vi "Startup.vi"(6 "LabVIEW Web Service":refnum<class "Web Service.lvclass">) -> ()   [LabVIEW 2017]
uses:
  <vilib>/wsapi/Web Service.lvclass
  <vilib>/NI_Real-Time Target Support.lvlib
panel:
  # "Use the web service input terminal to call the VIs on the Service subpalette of the Web Services palette. Do not remove it from the connector pane unless you don't need access to the palette."
  # "Any additional terminals added to the connector pane of a startup VI will be ignored."
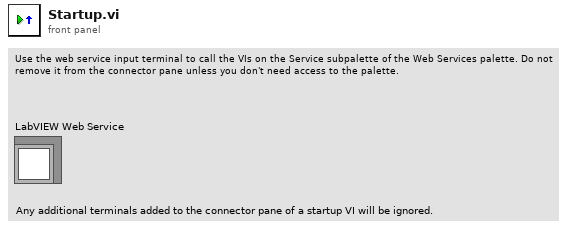
[diagram p1: front panel]
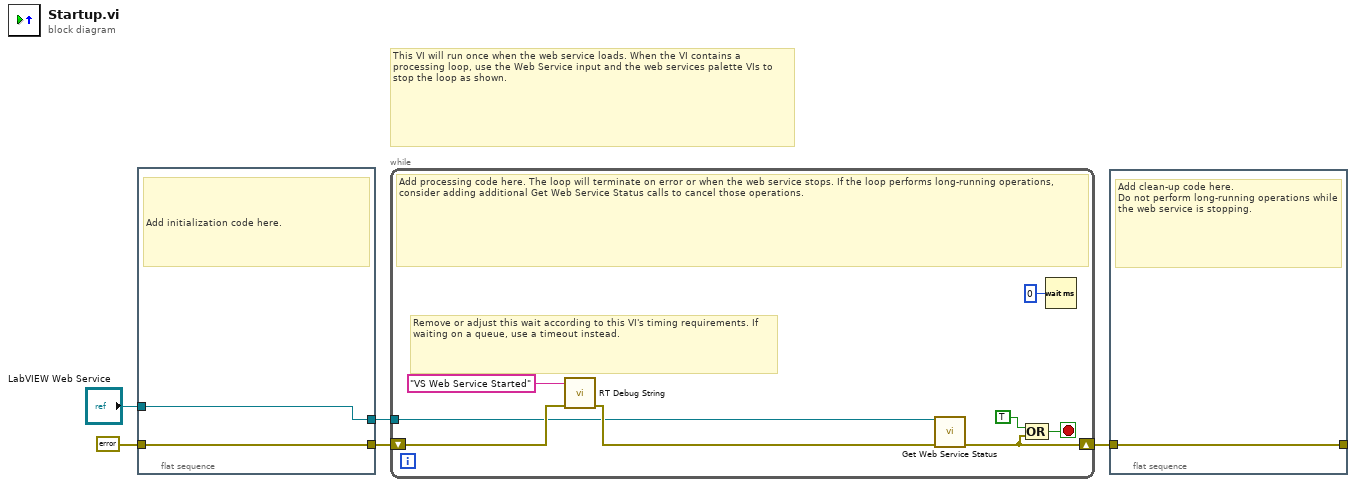
[diagram p0: block diagram]
diagram:
  # "This VI will run once when the web service loads. When the VI contains a processing loop, use the Web Service input and the web services palette VIs to stop the loop as shown."
  n1 = flat-sequence {
    tunnel: "LabVIEW Web Service" -> [w7]
    tunnel: [w7] -> w4
    tunnel: [w6] -> w3
    tunnel: errorcluster {"status"=FALSE, "code"=0, "source"=""} ("error constant") -> [w6]
    frame #0 {
      # "Add initialization code here."
    }
  }
  n2 = while {
    tunnel: w4 -> [w8]
    shift-right: [w13] -> w1
    shift-left: w3 -> [w11]
    stop <- w14 stop-if-true
    # "Remove or adjust this wait according to this VI's timing requirements. If waiting on a queue, use a timeout instead."
    # "Add processing code here. The loop will terminate on error or when the web service stops. If the loop performs long-running operations, consider adding additional Get Web Service Status calls to cancel those operations."
    n3 = call <vilib>:"RT Debug String.vi"("error in (no error)"=w11, "String to write"="VS Web Service Started") -> ("error out"=w10:errorcluster)  [unwired: 9 in]
    n4 = call <vilib>:"Get Web Service Status.vi"("LabVIEW Web Service"=w8, "error in (no error)"=w10) -> ("error out"=w13:errorcluster)  [unwired: 11 in, 2 out]
    n5 = Compound Arithmetic op=OR(TRUE, w13) -> (w14:bool)
    n6 = Wait (ms)(milliseconds to wait=u32 0) -> ()  [unwired: 1 out]
  }
  n7 = flat-sequence {
    tunnel: [w16] -> _
    tunnel: w1 -> [w16]
    frame #0 {
      # "Add clean-up code here.\nDo not perform long-running operations while the web service is stopping."
    }
  }
